vi "Write String.vi"(1 "Network Path":string, 3 "String":string, 4 "Tag Name":string) -> ()   [LabVIEW 2020]
uses:
  <vilib>/ethernetip/ethernetip.llb/EthernetIP Tag Write STRING.vi
  <vilib>/ethernetip/ethernetip.lvlib
panel:
  out "error out":errorcluster
  in  "error in":errorcluster
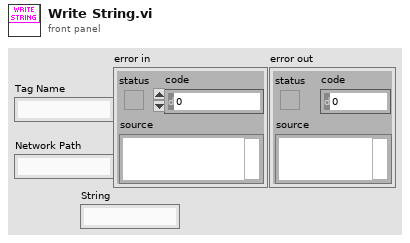
[diagram p1: front panel]
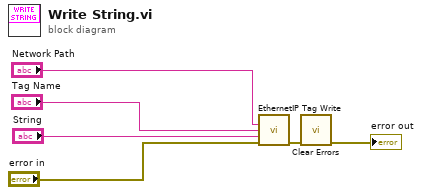
[diagram p0: block diagram]
diagram:
  n1 = call-poly <vilib>:"EthernetIP Tag Write.vi"("Network Path"="Network Path", "Tag Name"="Tag Name", "Data"="String", "error in"="error in") -> ("error out"=w3:errorcluster)  [unwired: 10 in, 1 out]
  n2 = call <vilib>:"Clear Errors.vi"("error in (no error)"=w3) -> ("error out"=→"error out":errorcluster)  [unwired: 5 in, 1 out]
